vi "Parse ppt document.vi"() -> ()   [LabVIEW 2014]
uses:
  DocumentFormat.OpenXml
panel:
  out "Array 4":string[][](array[string])
  out "Array":string[][](array[string])
  out "Array 2":string[][](array[string])
  out "Value":string[](array[string])
  out "InnerText":string[](array[string])
  out "HasValue":bool[](array[boolean])
  out "Slides":i32
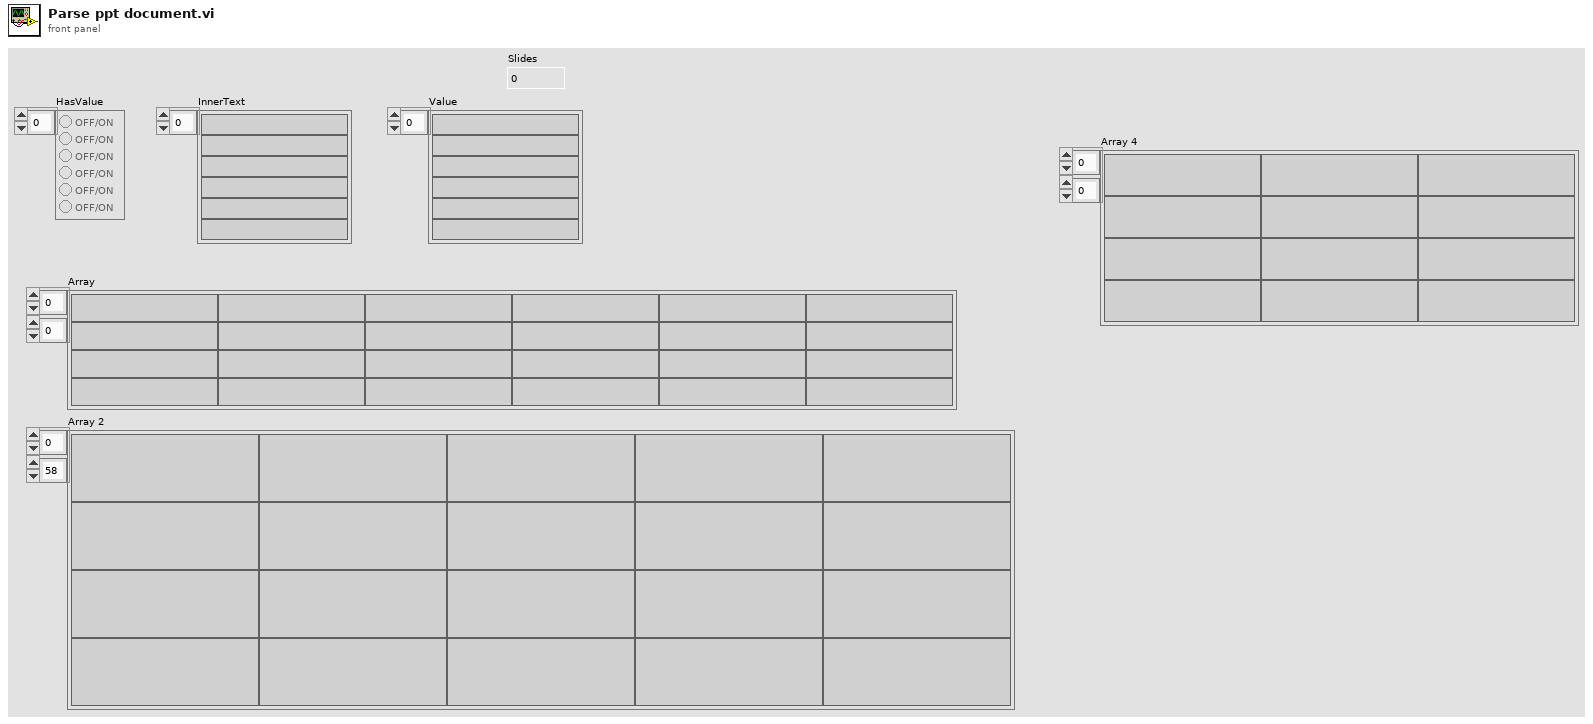
[diagram p1: front panel]
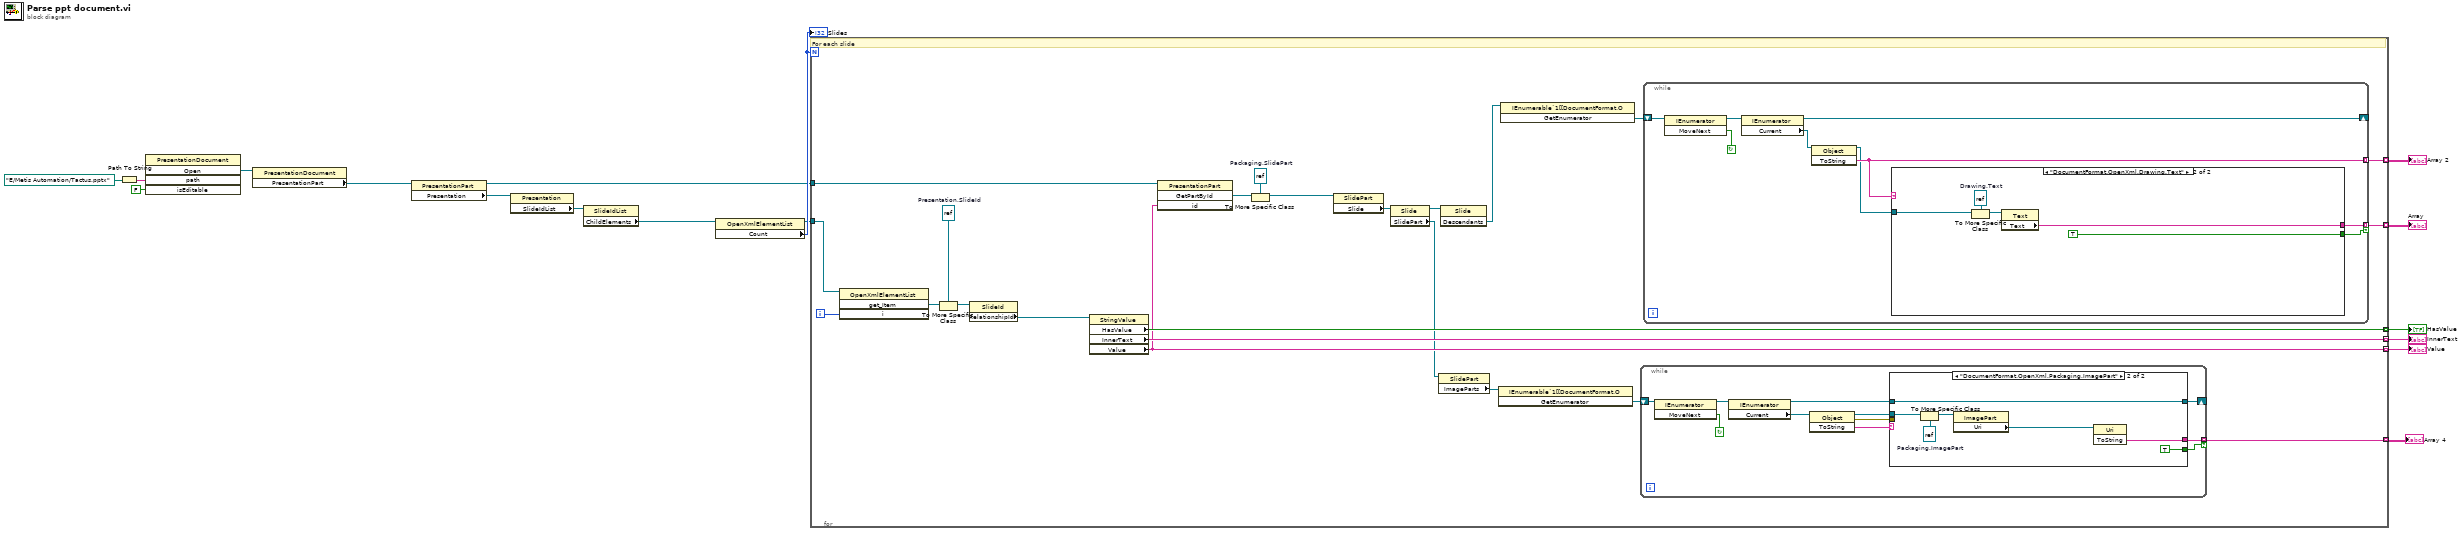
[diagram p0: block diagram]
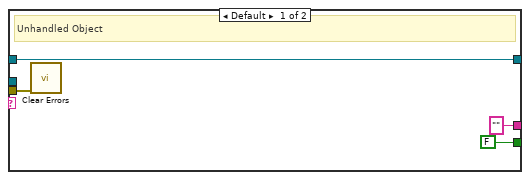
[diagram p2: hidden frame]
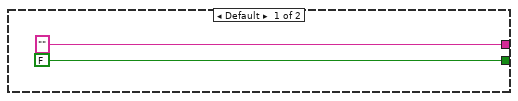
[diagram p3: hidden frame]
diagram:
  n1 = Path To String(path=path "E:/Metis Automation/Tactus.pptx") -> (string=w16:string)
  n2 = invoke class="PresentationDocument" method="Open"("path"=w16, "isEditable"=FALSE) -> ("Open"=w14:refnum<k24>)  [unwired: 3 in, 4 out]
  n3 = property class="PresentationDocument"(reference=w14) -> ("PresentationPart"=w13:refnum<k24>)  [unwired: 1 in, 2 out]
  n4 = property class="PresentationPart"(reference=w13) -> (reference out=w4:refnum<k24>, "Presentation"=w12:refnum<k24>)  [unwired: 1 in, 1 out]
  n5 = property class="Presentation"(reference=w12) -> ("SlideIdList"=w11:refnum<k24>)  [unwired: 1 in, 2 out]
  n6 = property class="SlideIdList"(reference=w11) -> ("ChildElements"=w10:refnum<k24>)  [unwired: 1 in, 2 out]
  n7 = property class="OpenXmlElementList"(reference=w10) -> (reference out=w8:refnum<k24>, "Count"=w9:i32)  [unwired: 1 in, 1 out]
  "Slides" <- w9
  n8 = for {
    N: w9 -> [_]
    tunnel: w8 -> [w40]
    tunnel: [w34] -> w7 mode=indexing
    tunnel: [w33] -> w6 mode=indexing
    tunnel: [w22] -> w5 mode=indexing
    tunnel: w4 -> [w32]
    tunnel: [w28] -> w3 mode=indexing
    tunnel: [w25] -> w2 mode=indexing
    tunnel: [w19] -> w1 mode=indexing
    i -> [w39]
    w30 = refnum<k24> refnum  # Packaging.SlidePart
    w36 = refnum<k24> refnum  # Presentation.SlideId
    # "For each slide"
    n9 = invoke class="OpenXmlElementList" method="get_Item"(reference=w40, "i"=w39) -> ("get_Item"=w38:refnum<k24>)  [unwired: 2 in, 3 out]
    n10 = To More Specific Class(target class=w36, reference=w38) -> (specific class reference=w37:refnum<k24>)  [unwired: 1 in, 1 out]
    n11 = property class="SlideId"(reference=w37) -> ("RelationshipId"=w35:refnum<k24>)  [unwired: 1 in, 2 out]
    n12 = property class="StringValue"(reference=w35) -> ("HasValue"=w34:bool, "InnerText"=w33:string, "Value"=w22:string)  [unwired: 1 in, 2 out]
    n13 = invoke class="PresentationPart" method="GetPartById"(reference=w32, "id"=w22) -> ("GetPartById"=w31:refnum<k24>)  [unwired: 2 in, 3 out]
    n14 = To More Specific Class(target class=w30, reference=w31) -> (specific class reference=w29:refnum<k24>)  [unwired: 1 in, 1 out]
    n15 = property class="SlidePart"(reference=w29) -> ("Slide"=w24:refnum<k24>)  [unwired: 1 in, 2 out]
    n16 = property class="Slide"(reference=w24) -> (reference out=w23:refnum<k24>, "SlidePart"=w21:refnum<k24>)  [unwired: 1 in, 1 out]
    n17 = property class="SlidePart"(reference=w21) -> ("ImageParts"=w18:refnum<k24>)  [unwired: 1 in, 2 out]
    n18 = invoke class="Slide" method="Descendants"(reference=w23) -> ("Descendants"=w26:refnum<k24>)  [unwired: 2 in, 2 out]
    n19 = invoke class="IEnumerable`1[[DocumentFormat.O" method="GetEnumerator"(reference=w18) -> ("GetEnumerator"=w20:refnum<k24>)  [unwired: 2 in, 2 out]
    n20 = invoke class="IEnumerable`1[[DocumentFormat.O" method="GetEnumerator"(reference=w26) -> ("GetEnumerator"=w27:refnum<k24>)  [unwired: 2 in, 2 out]
    n21 = while {
      shift-right: [w44] -> _
      shift-left: w20 -> [w51]
      tunnel: [w42] -> w19 mode=indexing if=w41
      stop <- w50 continue-if-true
      n22 = invoke class="IEnumerator" method="MoveNext"(reference=w51) -> (reference out=w49:refnum<k24>, "MoveNext"=w50:bool)  [unwired: 2 in, 1 out]
      n23 = property class="IEnumerator"(reference=w49) -> (reference out=w45:refnum<k24>, "Current"=w48:refnum<k24>)  [unwired: 1 in, 1 out]
      n24 = invoke class="Object" method="ToString"(reference=w48) -> (reference out=w43:refnum<k24>, error out=w46:errorcluster, "ToString"=w47:string)  [unwired: 2 in]
      n25 = case shown="\"DocumentFormat.OpenXml.Packaging.ImagePart\"" w47 {
        tunnel: w46 -> [w54 _]
        tunnel: w45 -> [w55 w62]
        tunnel: [w55 w62] -> w44
        tunnel: w43 -> [_ w60]
        tunnel: ["" ("AbsolutePath") w57] -> w42
        tunnel: [FALSE TRUE] -> w41
        frame Default {
          # "Unhandled Object"
          n26 = call <vilib>:"Clear Errors.vi"("error in (no error)"=w54) -> ()  [unwired: 5 in, 2 out]
        }
        frame "DocumentFormat.OpenXml.Packaging.ImagePart" {
          w61 = refnum<k24> refnum  # Packaging.ImagePart
          n27 = To More Specific Class(target class=w61, reference=w60) -> (specific class reference=w59:refnum<k24>)  [unwired: 1 in, 1 out]
          n28 = property class="ImagePart"(reference=w59) -> ("Uri"=w56:refnum<k24>)  [unwired: 1 in, 2 out]
          n29 = invoke class="Uri" method="ToString"(reference=w56) -> ("ToString"=w57:string)  [unwired: 2 in, 2 out]
        }
      }
    }
    n30 = while {
      shift-right: [w68] -> _
      shift-left: w27 -> [w71]
      tunnel: [w67] -> w28 mode=indexing
      tunnel: [w65] -> w25 mode=indexing if=w63
      stop <- w69 continue-if-true
      n31 = invoke class="IEnumerator" method="MoveNext"(reference=w71) -> (reference out=w70:refnum<k24>, "MoveNext"=w69:bool)  [unwired: 2 in, 1 out]
      n32 = property class="IEnumerator"(reference=w70) -> (reference out=w68:refnum<k24>, "Current"=w66:refnum<k24>)  [unwired: 1 in, 1 out]
      n33 = invoke class="Object" method="ToString"(reference=w66) -> (reference out=w64:refnum<k24>, "ToString"=w67:string)  [unwired: 2 in, 1 out]
      n34 = case shown="\"DocumentFormat.OpenXml.Drawing.Text\"" w67 {
        tunnel: w64 -> [_ w76]
        tunnel: ["" ("Text") w75] -> w65
        tunnel: [FALSE TRUE] -> w63
        frame Default {
        }
        frame "DocumentFormat.OpenXml.Drawing.Text" {
          w77 = refnum<k24> refnum  # Drawing.Text
          n35 = To More Specific Class(target class=w77, reference=w76) -> (specific class reference=w78:refnum<k24>)  [unwired: 1 in, 1 out]
          n36 = property class="Text"(reference=w78) -> ("Text"=w75:string)  [unwired: 1 in, 2 out]
        }
      }
    }
  }
  "HasValue" <- w7
  "InnerText" <- w6
  "Value" <- w5
  "Array 2" <- w3
  "Array" <- w2
  "Array 4" <- w1
